vi "Create.vi"(8 "error in":errorcluster, 11 "Type in":refnum<class "Type.lvclass">) -> (0 "error out":errorcluster, 3 "Type out":refnum<class "Type.lvclass">)   [LabVIEW 2020, in "_Rescript.lvlib" / "Type.lvclass"]
uses:
  Type.lvclass
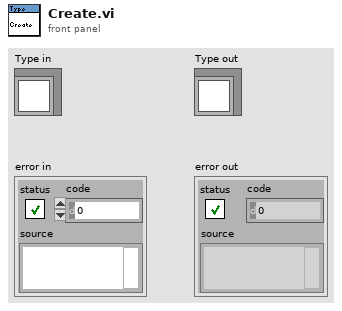
[diagram p1: front panel]
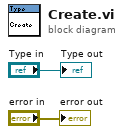
[diagram p0: block diagram]
diagram:
  "error out" <- "error in"
  "Type out" <- "Type in"
